vi "PDE_Sensor_Read_Setup (SubVI).vi"(8 "Error In":errorcluster, 9 "Pressure Freq":dbl, 10 "Temperature Freq":dbl, 11 "Sampling Time":dbl=1.0) -> (0 "error out":errorcluster, 1 "Samples Per Channel":dbl, 2 "Pressure Task":refnum<k21>, 3 "Temperature Task":refnum<k21>)   [LabVIEW 2016]
uses:
  <vilib>/DAQmx/create/channels.llb/DAQmx Create Channel (AI-Temperature-Thermocouple).vi
  <resource>/objmgr/daqmx.rc
  <vilib>/DAQmx/configure/timing.llb/DAQmx Timing (Sample Clock).vi
  <vilib>/DAQmx/create/channels.llb/DAQmx Create Channel (AI-Current-Basic).vi
  <vilib>/DAQmx/create/channels.llb/DAQmx Create Channel (AI-Voltage-Basic).vi
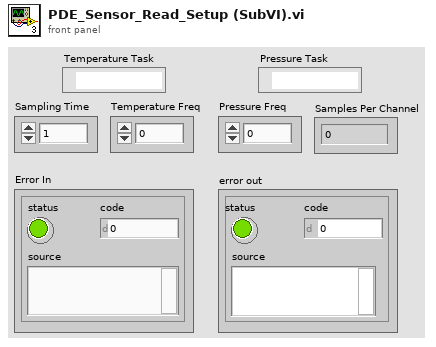
[diagram p1: front panel]
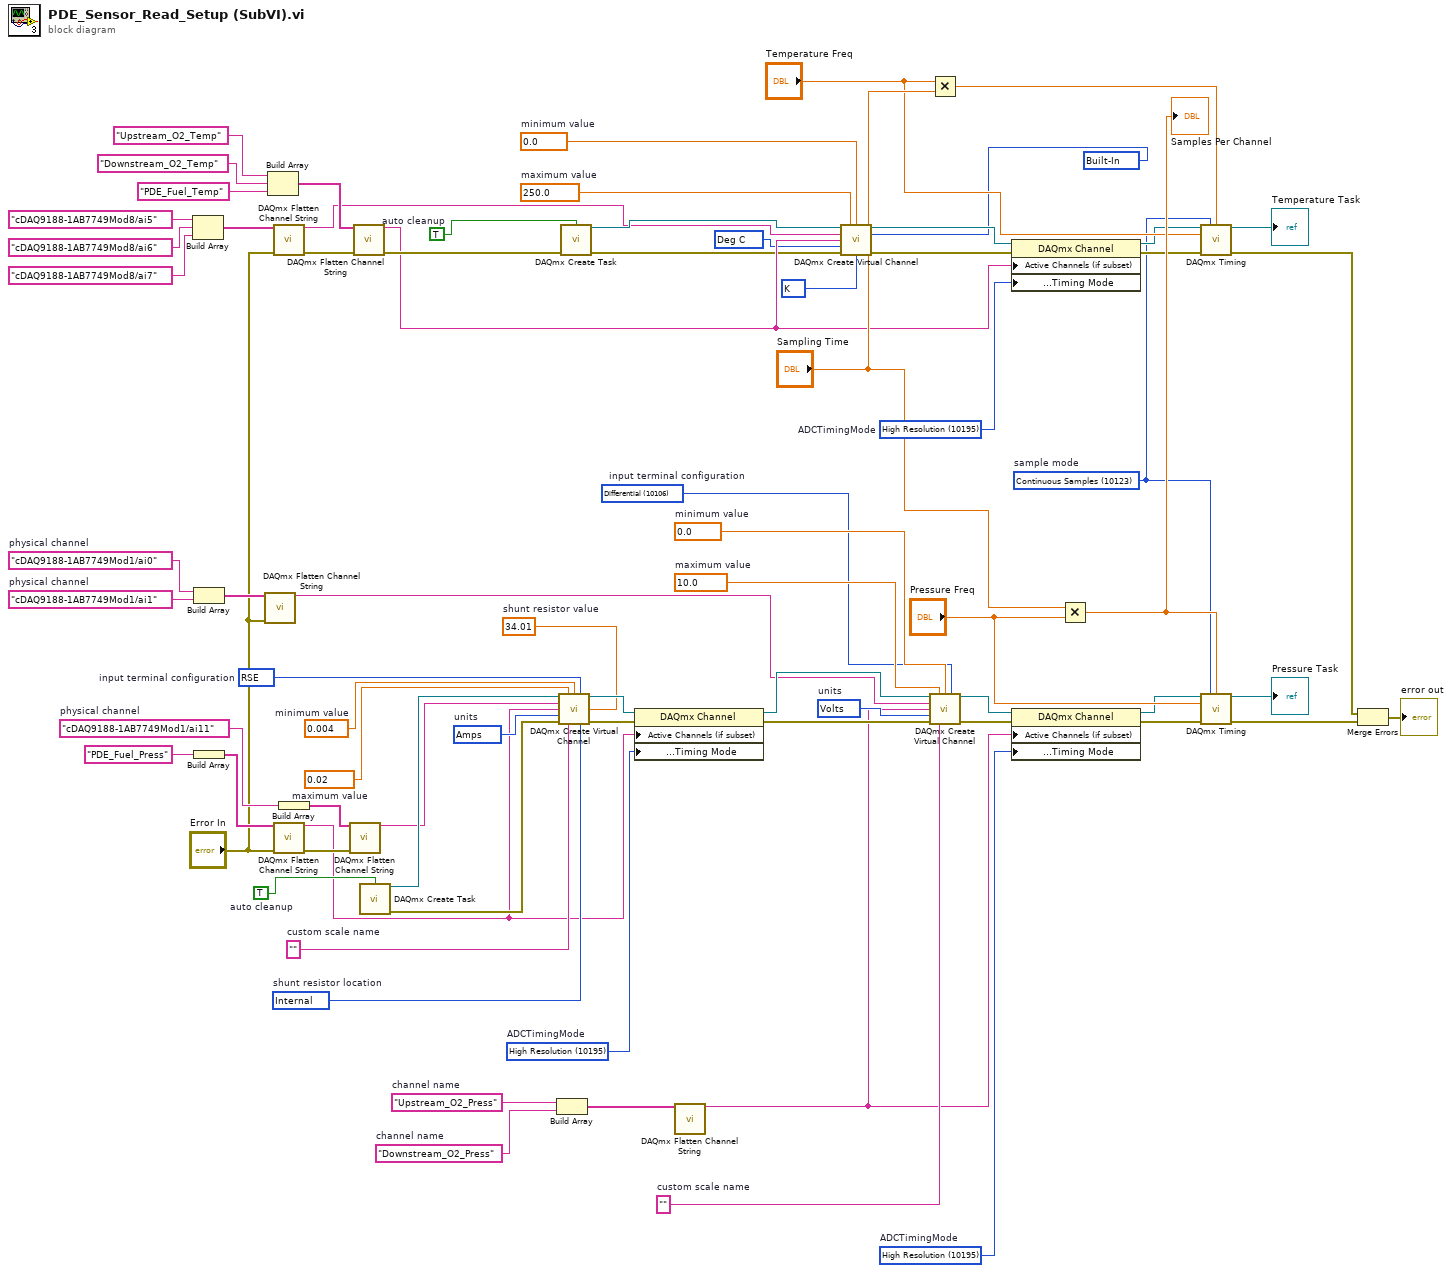
[diagram p0: block diagram]
diagram:
  w21 = 10195 items=["High Resolution"=10195, "High Speed"=14712, "Best 50 Hz Rejection"=14713, "Best 60 Hz Rejection"=14714]  # ADCTimingMode
  w10 = "Downstream_O2_Press"  # channel name
  w13 = "cDAQ9188-1AB7749Mod1/ai1"  # physical channel
  w22 = 10106 items=["default"=-1, "RSE"=10083, "NRSE"=10078, "Differential"=10106, "Pseudodifferential"=12529]  # input terminal configuration
  w8 = 10348 items=["Volts"=10348, "From Custom Scale"=10065]  # units
  w9 = "Upstream_O2_Press"  # channel name
  w23 = ""  # custom scale name
  w24 = 0.0  # minimum value
  w25 = 10.0  # maximum value
  w14 = "cDAQ9188-1AB7749Mod1/ai0"  # physical channel
  w27 = "cDAQ9188-1AB7749Mod1/ai11"  # physical channel
  w20 = 10123 items=["Finite Samples"=10178, "Continuous Samples"=10123, "Hardware Timed Single Point"=12522]  # sample mode
  w47 = 10195 items=["High Resolution"=10195, "High Speed"=14712, "Best 50 Hz Rejection"=14713, "Best 60 Hz Rejection"=14714]  # ADCTimingMode
  w46 = 10083 items=["default"=-1, "RSE"=10083, "NRSE"=10078, "Differential"=10106, "Pseudodifferential"=12529]  # input terminal configuration
  w45 = 10342 items=["Amps"=10342, "From Custom Scale"=10065]  # units
  w44 = 34.01  # shunt resistor value
  w43 = 10200 items=["Internal"=10200, "External"=10167]  # shunt resistor location
  w41 = ""  # custom scale name
  w40 = 0.004  # minimum value
  w39 = 0.02  # maximum value
  w37 = TRUE  # auto cleanup
  w51 = 10143 items=["Deg C"=10143, "Deg F"=10144, "Kelvins"=10325, "Deg R"=10145, "From Custom Scale"=10065] ("units")
  w52 = 10073 items=["J"=10072, "K"=10073, "N"=10077, "R"=10082, "S"=10085, "T"=10086, "B"=10047, "E"=10055] ("thermocouple type")
  w53 = 10200 items=["Built-In"=10200, "Constant Value"=10116, "Channel"=10113] ("cjc source")
  w62 = 10195 items=["High Resolution"=10195, "High Speed"=14712, "Best 50 Hz Rejection"=14713, "Best 60 Hz Rejection"=14714]  # ADCTimingMode
  w59 = 0.0  # minimum value
  w58 = 250.0  # maximum value
  w56 = TRUE  # auto cleanup
  n1 = Build Array("cDAQ9188-1AB7749Mod8/ai5" ("element"), "cDAQ9188-1AB7749Mod8/ai6" ("element"), "cDAQ9188-1AB7749Mod8/ai7" ("element")) -> (w50:string[])
  n2 = Build Array(w14, w13) -> (w15:string[])
  n3 = Build Array("PDE_Fuel_Press" ("element")) -> (w34:string[])
  n4 = call <vilib>:"DAQmx Flatten Channel String.vi"("names in"=w15, "error in"="Error In") -> ("names out"=w12:string)  [unwired: 12 in, 1 out]
  n5 = Build Array("Upstream_O2_Temp" ("name to assign"), "Downstream_O2_Temp" ("name to assign"), "PDE_Fuel_Temp" ("name to assign")) -> (w65:string[])
  n6 = call <vilib>:"DAQmx Flatten Channel String.vi"("names in"=w50, "error in"="Error In") -> ("names out"=w54:string, "error out"=w77:errorcluster)  [unwired: 12 in]
  n7 = call <vilib>:"DAQmx Flatten Channel String.vi"("names in"=w34, "error in"="Error In") -> ("names out"=w33:string, "error out"=w76:errorcluster)  [unwired: 12 in]
  n8 = Build Array(w27) -> (w32:string[])
  n9 = call <vilib>:"DAQmx Flatten Channel String.vi"("names in"=w32, "error in"=w76) -> ("names out"=w35:string)  [unwired: 12 in, 1 out]
  n10 = call <vilib>:"DAQmx Flatten Channel String.vi"("names in"=w65, "error in"=w77) -> ("names out"=w69:string, "error out"=w70:errorcluster)  [unwired: 12 in]
  n11 = call <vilib>:"DAQmx Create Task.vi"("auto cleanup"=w37) -> ("task out"=w38:refnum<k21>, "error out"=w36:errorcluster)  [unwired: 4 in, 9 out]
  n12 = Build Array(w9, w10) -> (w11:string[])
  n13 = call-poly <vilib>:"DAQmx Create Virtual Channel.vi"("task in"=w38, "maximum value"=w39, "minimum value"=w40, "input terminal configuration"=w46, "physical channels"=w35, "name to assign"=w33, "external shunt resistor value"=w44, "units"=w45, "error in"=w36, "custom scale name"=w41, "shunt resistor location"=w43) -> ("task out"=w48:refnum<k21>, "error out"=w42:errorcluster)  [unwired: 3 out]
  n14 = call <vilib>:"DAQmx Create Task.vi"("auto cleanup"=w56, "error in"=w70) -> ("task out"=w57:refnum<k21>, "error out"=w55:errorcluster)  [unwired: 3 in, 9 out]
  n15 = property class="DAQmx Channel"(reference=w48, error in=w42, "Active Channels (if subset)"=w33, "Analog Input:General Properties:Digitizer/ADC:Timing Mode"=w47) -> (reference out=w18:refnum<k21>, error out=w17:errorcluster)
  n16 = call <vilib>:"DAQmx Flatten Channel String.vi"("names in"=w11) -> ("names out"=w5:string)  [unwired: 13 in, 1 out]
  n17 = call-poly <vilib>:"DAQmx Create Virtual Channel.vi"("task in"=w57, "maximum value"=w58, "minimum value"=w59, "physical channels"=w54, "cjc source"=w53, "name to assign"=w69, "units"=w51, "error in"=w55, "thermocouple type"=w52) -> ("task out"=w63:refnum<k21>, "error out"=w60:errorcluster)  [unwired: 5 in]
  n18 = Multiply(x="Temperature Freq", y="Sampling Time") -> (x*y=w73:dbl)
  n19 = call-poly <vilib>:"DAQmx Create Virtual Channel.vi"("task in"=w18, "maximum value"=w25, "minimum value"=w24, "input terminal configuration"=w22, "physical channels"=w12, "name to assign"=w5, "units"=w8, "error in"=w17, "custom scale name"=w23) -> ("task out"=w7:refnum<k21>, "error out"=w6:errorcluster)  [unwired: 5 in]
  n20 = property class="DAQmx Channel"(reference=w63, error in=w60, "Active Channels (if subset)"=w69, "Analog Input:General Properties:Digitizer/ADC:Timing Mode"=w62) -> (reference out=w64:refnum<k21>, error out=w61:errorcluster)
  n21 = property class="DAQmx Channel"(reference=w7, error in=w6, "Active Channels (if subset)"=w5, "Analog Input:General Properties:Digitizer/ADC:Timing Mode"=w21) -> (reference out=w19:refnum<k21>, error out=w16:errorcluster)
  n22 = Multiply(x="Sampling Time", y="Pressure Freq") -> (x*y=w74:dbl)
  "Samples Per Channel" <- w74
  n23 = call-poly <vilib>:"DAQmx Timing.vi"("task/channels in"=w64, "sample mode"=w20, "samples per channel"=w73, "rate"="Temperature Freq", "error in"=w61) -> ("task out"=→"Temperature Task":refnum<k21>, "error out"=w2:errorcluster)  [unwired: 2 in, 7 out]
  n24 = call-poly <vilib>:"DAQmx Timing.vi"("task/channels in"=w19, "sample mode"=w20, "samples per channel"=w74, "rate"="Pressure Freq", "error in"=w16) -> ("task out"=→"Pressure Task":refnum<k21>, "error out"=w4:errorcluster)  [unwired: 2 in, 7 out]
  n25 = Merge Errors(w2, w4) -> (→"error out":errorcluster)
